vi "Clear quench.vi"(8 "error in (no error)":errorcluster, 11 "PS Driver AMI4xx in":refnum<class "PS Driver AMI4xx.lvclass">) -> (0 "error out":errorcluster, 3 "PS Driver AMI4xx out":refnum<class "PS Driver AMI4xx.lvclass">)   [LabVIEW 2025, in "PS Driver.lvlib" / "PS Driver AMI4xx.lvclass"]
doc: "Author: Scott Hannahs <sth@magnet.fsu.edu>\n\nThis software is licensed for use under the “MIT License\"\nCopyright (c) 2025 Scott Hannahs, sth@sth@magnet.sthnet.net\n\nPermission is hereby granted, free of charge, to any person obtaining a copy of this software and associated documentation files (the \"Software\"), to deal in the Software without restriction, including without limitation the rights to use, copy, modify, merge, publish, distribute, sublicense, and/or sell copies of the Software, and to permit persons to whom the Software is furnished to do so, subject to the following conditions: The above copyright notice and this permission notice shall be included in all copies or substantial portions of the Software.\n\nTHE SOFTWARE IS PROVIDED \"AS IS\", WITHOUT WARRANTY OF ANY KIND, EXPRESS OR IMPLIED, INCLUDING BUT NOT LIMITED TO THE WARRANTIES OF MERCHANTABILITY, FITNESS FOR A PARTICULAR PURPOSE AND NONINFRINGEMENT. IN NO EVENT SHALL THE AUTHORS OR COPYRIGHT HOLDERS BE LIABLE FOR ANY CLAIM, DAMAGES OR OTHER LIABILITY, WHETHER IN AN ACTION OF CONTRACT, TORT OR OTHERWISE, ARISING FROM, OUT OF OR IN CONNECTION WITH THE SOFTWARE OR THE USE OR OTHER DEALINGS IN THE SOFTWARE."
uses:
  PS Driver AMI4xx.lvclass
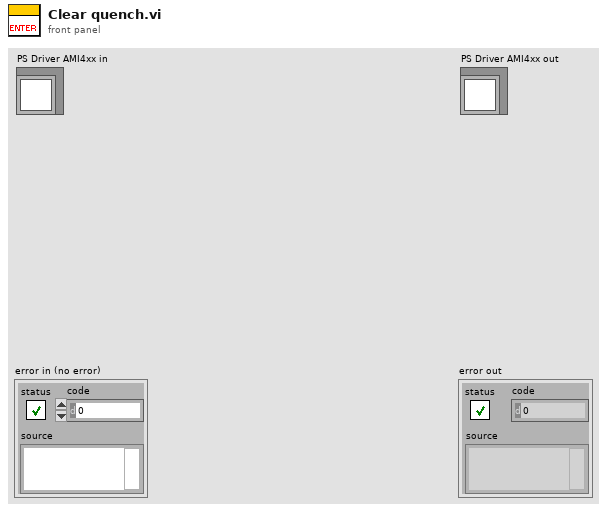
[diagram p1: front panel]
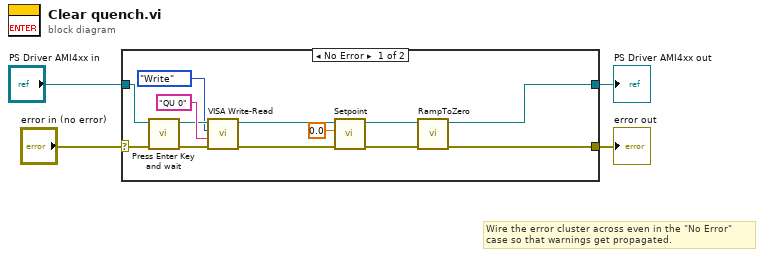
[diagram p0: block diagram]
diagram:
  # "Wire the error cluster across even in the \"No Error\"\ncase so that warnings get propagated."
  n1 = case shown="No Error" "error in (no error)" {
    selector: "error in (no error)" -> [w15 w19]
    tunnel: [w9 w19] -> w3
    tunnel: [w7 w18] -> w1
    tunnel: "PS Driver AMI4xx in" -> [w14 w18]
    frame No Error {
      n2 = call "Press Enter Key and wait.vi"("error in (no error)"=w15, "PS Driver AMI4xx in"=w14) -> ("error out"=w16:errorcluster, "PS Driver AMI4xx out"=w13:refnum<class "PS Driver AMI4xx.lvclass">)  [unwired: 8 in]
      n3 = call "VISA Write-Read.vi"("error in (no error)"=w16, "Command String"="QU 0", "Action"=enum16{"Write", "Read", "Write & Read"}."Write", "PS Driver.lvlib:PS Driver AMI4xx.lvclass"=w13) -> ("error out"=w11:errorcluster, "PS Driver.lvlib:PS Driver AMI4xx.lvclass out"=w6:refnum<class "PS Driver AMI4xx.lvclass">)  [unwired: 4 in, 2 out]
      n4 = call-dynamic "Setpoint.vi"("error in (no error)"=w11, "Setpoint [A]"=0.0, "PS Driver AMI4xx.lvlib:PS Driver AMI4xx.lvclass in"=w6) -> ("error out"=w10:errorcluster, "PS Driver AMI4xx.lvlib:PS Driver AMI4xx.lvclass out"=w8:refnum<class "PS Driver AMI4xx.lvclass">)  [unwired: 6 in, 1 out]
      n5 = call-dynamic "RampToZero.vi"("error in (no error)"=w10, "PS Driver AMI4xx.lvlib:PS Driver AMI4xx.lvclass in"=w8) -> ("error out"=w9:errorcluster, "PS Driver AMI4xx.lvlib:PS Driver AMI4xx.lvclass out"=w7:refnum<class "PS Driver AMI4xx.lvclass">)  [unwired: 8 in]
    }
    frame Error {
    }
  }
  "error out" <- w3
  "PS Driver AMI4xx out" <- w1
